vi "Get Fields for Searching.vi"(8 "error in":errorcluster) -> (0 "error out":errorcluster, 1 "Serial Number":string, 2 "Model Number":string, 3 "Field Records List":string[](array[string]))   [LabVIEW 2011]
uses:
  typedefs/Field Order By.ctl
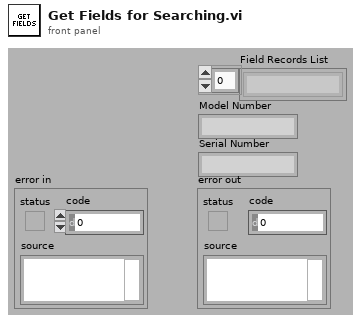
[diagram p1: front panel]
types:
  T1 = typedef "Field Order By.ctl" = enum32{"sxSequenceId", "sxFieldId", "sDisplayName", "sValue", "fSetAtTest", "fRequired", "nNextItem"}
  T2 = typedef "Connection Refnum.ctl" = cluster{"Environment Handle":i32, "Connection Handle":i32}
  T3 = typedef "Field Record.ctl" = cluster{"ixField":i32, "iSequenceOrder":i32, "sxFieldId":string, "sxSequenceId":string, "sDisplayName":string, "sValue":string, "sUnits":string, "nDataType":T4, "nNextItem":T5, "fSystem":bool, "fSystemValue":bool, "fRequired":bool, "fSetAtTest":bool, "fTestField":bool, "fDeleted":bool, "fIndexed":bool, "fFreeList":bool}
  T4 = typedef "Field DataTypes.ctl" = enum32{"text", "numeric", "list", "timestamp", "boolean"}
  T5 = typedef "Field NextItem.ctl" = enum32{"Reset", "Retain", "Auto-Increment"}
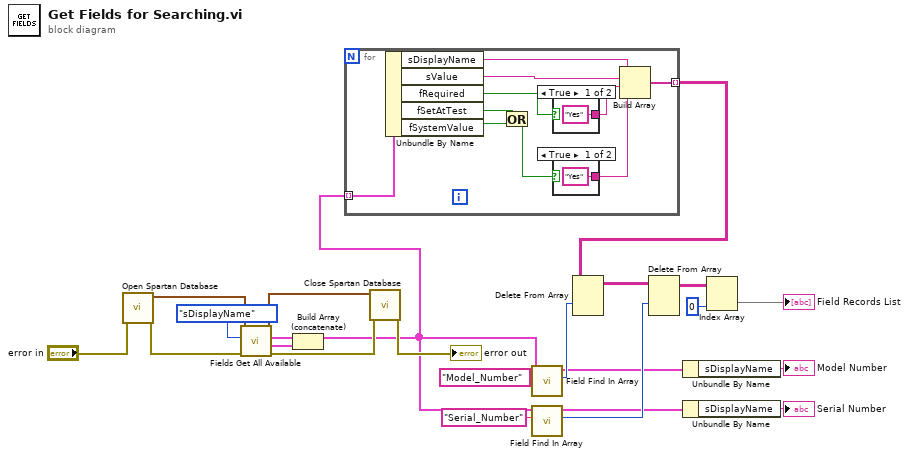
[diagram p0: block diagram]
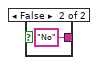
[diagram p2: hidden frame]
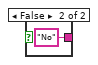
[diagram p3: hidden frame]
diagram:
  n1 = call "Open Spartan Database.vi"("error in (no error)"="error in") -> ("error out"=w9:errorcluster, "Connection Refnum"=w8:T2)  [unwired: 1 in, 8 out]
  n2 = call "Fields Get All Available.vi"("error in (no error)"=w9, "Sort by (sxSequenceId)"=Field_Order_By."sDisplayName" ("Sort by (Sequence_ID)"), "Connection Refnum"=w8) -> ("error out"=w7:errorcluster, "Custom Fields"=w3:T3[], "System or ALL Combined Fields"=w4:T3[], "Connection Refnum"=w5:T2)  [unwired: 2 in, 3 out]
  n3 = Build Array (concatenate)(w4, w3) -> (w2:T3[])
  n4 = for {
    tunnel: [w33] -> w1 mode=indexing
    tunnel: w2 -> [w30] mode=indexing
    n5 = Unbundle By Name(w30) -> ("sDisplayName"=w29:string, "sValue"=w28:string, "fRequired"=w27:bool, "fSetAtTest"=w26:bool, "fSystemValue"=w25:bool)
    n6 = Or(x=w26, y=w25) -> (x .or. y?=w24:bool)
    n7 = case shown="True" w27 {
      tunnel: ["Yes" "No"] -> w32
      frame True {
      }
      frame False {
      }
    }
    n8 = case shown="True" w24 {
      tunnel: ["Yes" "No"] -> w31
      frame True {
      }
      frame False {
      }
    }
    n9 = Build Array(w29, w28, w32, w31) -> (w33:string[])
  }
  n10 = call "Close Spartan Database.vi"("error in (no error)"=w7, "Connection Refnum"=w5) -> ("error out"=→"error out":errorcluster)  [unwired: 2 in, 7 out]
  n11 = call "Field Find In Array.vi"("FieldID or Display Name(\"\")"="Model_Number" ("Field_ID (\"\")"), "Field Array"=w2) -> ("Index"=w18:i32, "Field"=w14:T3)  [unwired: 1 in, 7 out]
  n12 = call "Field Find In Array.vi"("FieldID or Display Name(\"\")"="Serial_Number" ("Field_ID (\"\")"), "Field Array"=w2) -> ("Index"=w17:i32, "Field"=w13:T3)  [unwired: 1 in, 7 out]
  n13 = Delete From Array(array=w1, index (row)=w18) -> (array with subset deleted=w16:string[][])  [unwired: 2 in, 1 out]
  n14 = Delete From Array(array=w16, index (row)=w17) -> (array with subset deleted=w15:string[][])  [unwired: 2 in, 1 out]
  n15 = Unbundle By Name(w14) -> ("sDisplayName"=→"Model Number":string)
  n16 = Unbundle By Name(w13) -> ("sDisplayName"=→"Serial Number":string)
  n17 = Index Array(array=w15, index (col)=0 ("disabled index (col)")) -> (element=→"Field Records List":string[])  [unwired: 1 in]
